vi "Edit Configuration File.vi"(11 "error in (no error)":errorcluster) -> (15 "error out":errorcluster)   [LabVIEW 2021]
uses:
  <vilib>/Utility/sysdir.llb/System Directory Type.ctl
  <vilib>/Utility/config.llb/Write Key (String).vi
  <vilib>/Utility/config.llb/NI_LVConfig.lvlib
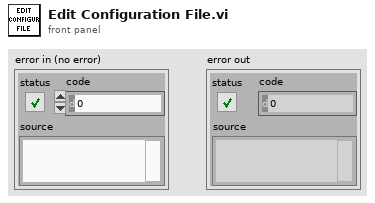
[diagram p1: front panel]
types:
  T1 = typedef "System Directory Type.ctl" = i32
  T2 = typedef "NI_LVConfig.lvlib/Config Data RefNum.ctl" = refnum<k1>
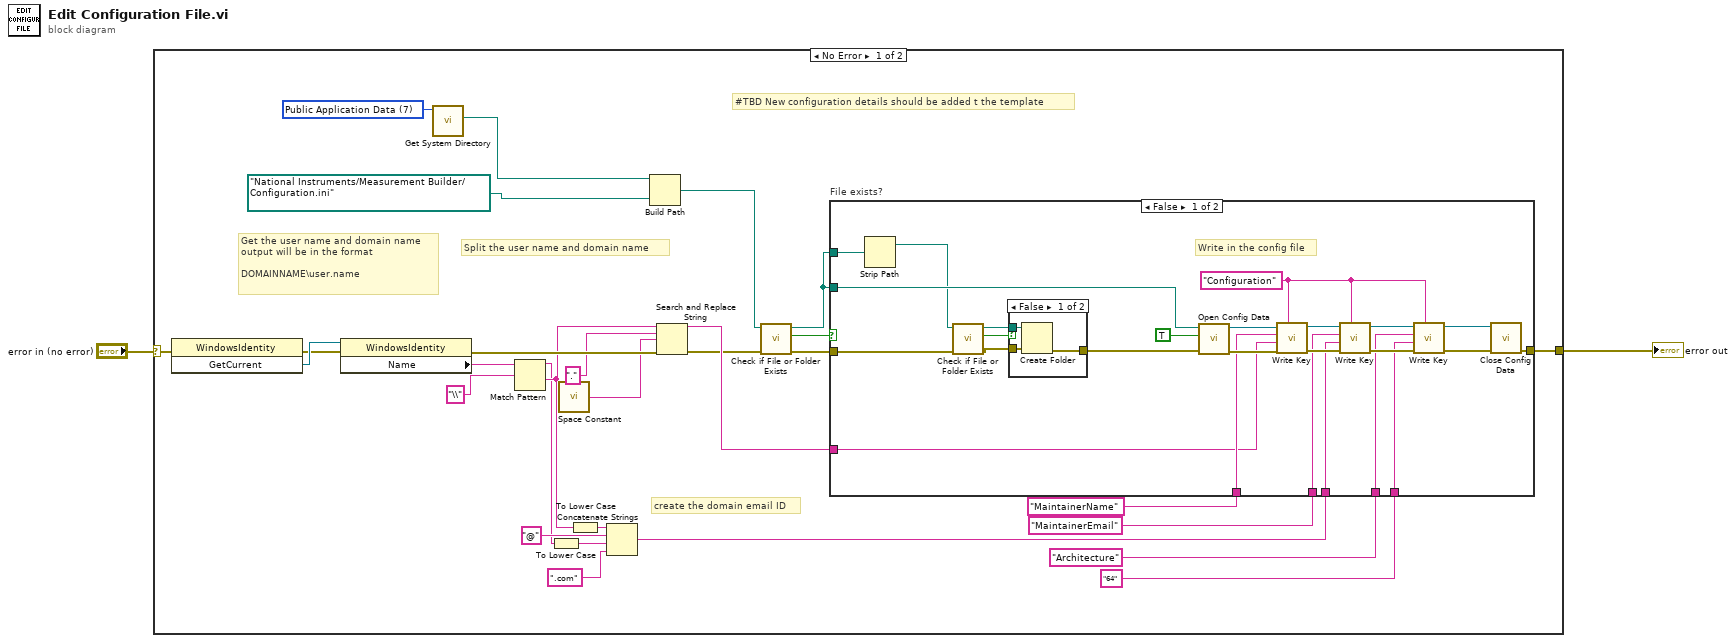
[diagram p0: block diagram]
diagram:
  n1 = case shown="No Error" "error in (no error)" {
    selector: "error in (no error)" -> [w27 w62]
    tunnel: [w31 w62] -> w1
    frame No Error {
      w10 = T1 7 items=["User Home"=0, "User Desktop"=1, "User Documents"=2, "User Application Data"=3, "User Preferences"=4, "User Temporary"=5, "Public Documents"=6, "Public Application Data"=7, "Public Preferences"=8, "Public Cache"=13, "System Core Libraries"=9, "System Installed Libraries"=10, "Application Files"=11, "Boot Volume Root"=12] ("system directory type")
      # "#TBD New configuration details should be added t the template"
      # "create the domain email ID"
      # "Split the user name and domain name"
      # "Get the user name and domain name\noutput will be in the format\n\nDOMAINNAME\\user.name"
      n2 = invoke class="WindowsIdentity" method="GetCurrent"(error in=w27) -> (error out=w26:errorcluster, "GetCurrent"=w30:refnum<k24>)  [unwired: 2 in, 1 out]
      n3 = property class="WindowsIdentity"(reference=w30, error in=w26) -> (error out=w25:errorcluster, "Name"=w28:string)  [unwired: 1 out]
      n4 = call <vilib>:"Get System Directory.vi"("system directory type"=w10) -> ("system directory"=w9:path)  [unwired: 10 in]
      n5 = Match Pattern(string=w28, regular expression="\\") -> (before substring=w18:string, after substring=w20:string)  [unwired: 1 in, 2 out]
      n6 = To Lower Case(string=w18) -> (all lower case string=w17:string)
      n7 = call <vilib>:"Space Constant.vi"() -> ("String"=w23:string)
      n8 = To Lower Case(string=w20) -> (all lower case string=w7:string)
      n9 = Concatenate Strings(w7, "@" ("string"), w17, ".com" ("string")) -> (w15:string)
      n10 = Build Path(base path=w9, name or relative path=path "National Instruments/Measurement Builder/Configuration.ini") -> (appended path=w4:path)
      n11 = Search and Replace String(input string=w20, search string=".", replace string=w23, error in=w25) -> (result string=w14:string, error out=w12:errorcluster)  [unwired: 4 in, 2 out]
      n12 = call <vilib>:"Check if File or Folder Exists.vi"("error in (no error)"=w12, "path"=w4) -> ("error out"=w13:errorcluster, "file or folder exists?"=w11:bool, "dup path"=w3:path)  [unwired: 7 in]
      n13 = case "File exists?" shown="False" w11 {
        tunnel: [w52 w61] -> w31
        tunnel: "MaintainerName" ("section") -> [w51 _]
        tunnel: "MaintainerEmail" ("section") -> [w50 _]
        tunnel: w15 -> [w49 _]
        tunnel: w14 -> [w48 _]
        tunnel: w3 -> [w47 _]
        tunnel: w13 -> [w34 w61]
        tunnel: "Architecture" ("section") -> [w40 _]
        tunnel: "64" ("section") -> [w39 _]
        tunnel: w3 -> [w38 _]
        frame False {
          w41 = "Configuration" ("section")
          # "Write in the config file"
          n14 = Strip Path(path=w38) -> (stripped path=w37:path)  [unwired: 1 out]
          n15 = call <vilib>:"Check if File or Folder Exists.vi"("error in (no error)"=w34, "path"=w37) -> ("error out"=w35:errorcluster, "file or folder exists?"=w36:bool, "dup path"=w32:path)  [unwired: 7 in]
          n16 = case shown="False" w36 {
            tunnel: w35 -> [w59 w60]
            tunnel: [w58 w60] -> w33
            tunnel: w32 -> [w57 _]
            frame False {
              n17 = Create Folder(path (use dialog)=w57, error in=w59) -> (error out=w58:errorcluster)  [unwired: 1 in, 2 out]
            }
            frame True {
            }
          }
          n18 = call <vilib>:"Open Config Data.vi"("error in (no error)"=w33, "create file if necessary (T)"=TRUE, "configuration file path"=w47) -> ("error out"=w56:errorcluster, "refnum"=w55:T2)  [unwired: 6 in, 1 out]
          n19 = call-poly <vilib>:"Write Key.vi"("section"=w41, "error in (no error)"=w56, "value"=w48, "key"=w51, "refnum"=w55) -> ("error out"=w54:errorcluster, "refnum out"=w53:T2)  [unwired: 4 in, 1 out]
          n20 = call-poly <vilib>:"Write Key.vi"("section"=w41, "error in (no error)"=w54, "value"=w49, "key"=w50, "refnum"=w53) -> ("error out"=w43:errorcluster, "refnum out"=w45:T2)  [unwired: 4 in, 1 out]
          n21 = call-poly <vilib>:"Write Key.vi"("section"=w41, "error in (no error)"=w43, "value"=w39, "key"=w40, "refnum"=w45) -> ("error out"=w42:errorcluster, "refnum out"=w44:T2)  [unwired: 4 in, 1 out]
          n22 = call <vilib>:"Close Config Data.vi"("error in (no error)"=w42, "refnum"=w44) -> ("error out"=w52:errorcluster)  [unwired: 8 in, 1 out]
        }
        frame True {
        }
      }
    }
    frame Error {
    }
  }
  "error out" <- w1
